vi "editDialog.vi"(0 "reference":refnum<class "ClassNode.lvclass">, 1 "insidePackageNode":bool, 5 "error in (no error)":errorcluster) -> (14 "reference out":refnum<class "ClassNode.lvclass">, 15 "changeConnection":T2, 16 "cancel":bool, 19 "error out":errorcluster)   [LabVIEW 2016, in "ClassNode.lvclass"]
doc: "Edit Dialog"
uses:
  <resource>/Framework/Providers/Open_GDS/UML/ClassNode_class/ClassNode.lvclass
  C:/Program Files (x86)/National Instruments/LabVIEW 2016/resource/Framework/Providers/Open_GDS/UML/AbstractNode_class/AbstractNode.lvclass
  <resource>/Framework/Providers/Open_GDS/UML/AbstractNode_class/private/NodeConnectionStatsType.ctl
  <resource>/Framework/Providers/Open_GDS/UML/UMLEditor/UMLEditor_StoredPathes.ctl
  <resource>/Framework/Providers/Open_GDS/ClassProviders/Common/CommonVIs/CommonVIs_StereoType.ctl
  <resource>/Framework/Providers/Open_GDS/UML/ContextHelp/ContextHelp_HelpTexts.ctl
  <resource>/Framework/Providers/Open_GDS/UML/MultiLineString_class/MultiLineString.lvclass
  <resource>/Framework/Providers/Open_GDS/UML/AbstractNode_class/AbstractNode.lvclass
  <resource>/Framework/Providers/Open_GDS/UML/Graph_class/Graph.lvclass
panel:
  in  "Class owner":u16(ring) items=["<No owner>", "FalconRocket", "RocketEngineBase", "SimulatedRocket", "TempSensor", "TestSystem"]
  out "RelText":string="Relative path used"
  out "UserText":string="When creating an enum-type just state the different enumeration members in a list like this:\nE.g.\nElement 1\nElement 2\n\nE.g.\nVolt(V)\nCurrent(A)\nResistance(ohm)\n"
  in  "ShowAttrib":bool caption="Show Attributes"
  in  "ShowMethods":bool caption="Show Methods"
  in  "Help":bool
  in  "AddMethod":bool
  in  "AddAttribute":bool
  in  "Stereo Type":T1(ring)=enum."ENUM"
  in  "Class Name":string
  in  "ClassPath":path caption="LvClassPath(Optional)"
  in  "Attribute":string
  in  "Methods":string
  in  "connection":bool caption="Connect to Package"
  in  "Cancel Button":bool
  in  "OK Button":bool
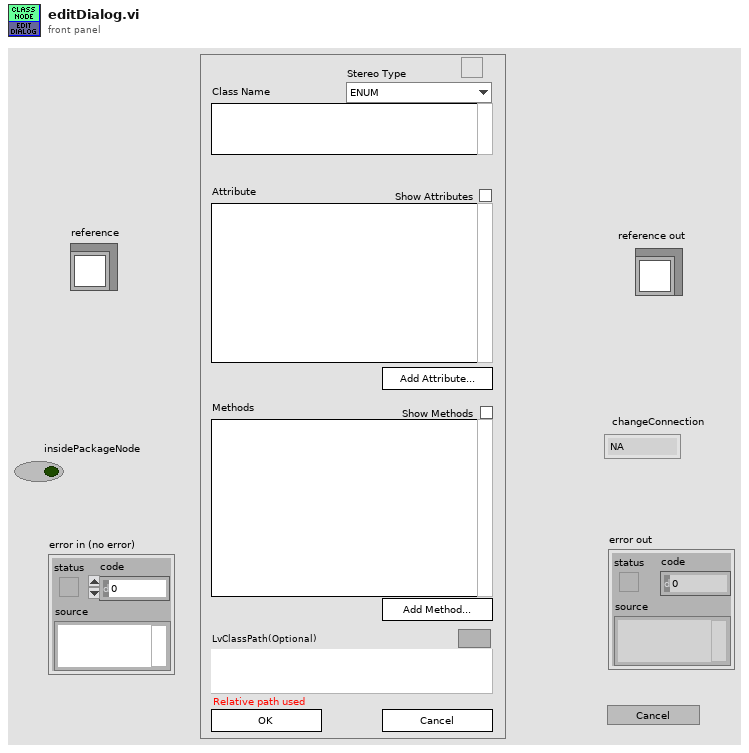
[diagram p1: front panel]
types:
  T1 = enum16{"None", "TYPE", "ENUM", "ABSTRACT", "ACTOR", "GUI", "SINGLETON", "SIGNAL", "BOUNDARY", "ENTITY", "CONTROL", "LEGACY", "APPLICATION", "VI", "LVLIB"}
  T2 = typedef "AbstractNode.lvclass/NodeConnectionStatsType.ctl" = enum16{"NA", "Connect", "DisConnect"}
  T3 = typedef "CommonVIs_StereoType.ctl" = enum16{"None", "TYPE", "ENUM", "ABSTRACT", "ACTOR", "GUI", "SINGLETON", "SIGNAL", "BOUNDARY", "ENTITY", "CONTROL", "LEGACY", "APPLICATION", "VI", "LVLIB"}
  T4 = typedef "UMLEditor_StoredPathes.ctl" = enum16{"LastSearchPath", "QueuedArrayStateVI", "ClassBasePath", "ViTemplatePath", "ApplicationTemplatePath", "IniFilePath", "WizDir", "RevPlugInPath"}
  T5 = enum32{"existing file", "new file", "new or existing file", "existing dir", "new dir", "new or existing dir", "existing file (use LLBs)", "new file (use LLBs)", "new or existing file (use LLBs)", "new or existing file or directory (use LLBs)"}
  T6 = enum16{"None", "TYPE", "ENUM", "GUI", "SINGLETON", "SIGNAL", "BOUNDARY", "ENTITY", "CONTROL", "LEGACY", "APPLICATION", "VI", "LVLIB"}
  T7 = typedef "ContextHelp_HelpTexts.ctl" = enum16{"None(Hide)", "Default", "Help", "Welcome", "GettingStarted", "ClassDiagram_Help", "SequenceDiagram_Help", "UseCaseDiagram_Help", "BSelect", "BClass", "BInterface", "BPackage", "BNote", "BDependency", "BInheritance", "BInterfaceImplementation", "BAssociation", "BAggregation", "BCompAggregation", "BNoteConnector", "BObject", "BActionBar", "BCall", "BSystem", "BActor", "BUseCase", "BGeneralization", "BIncludes", "BExtends", "BUseCaseDiagramAssociation", "ClassRelationshipEdge editDialog_Bent Style", "ClassRelationshipEdge editDialog_RelationType", "ClassRelationshipEdge editDialog_Reverse association", "ClassRelationshipEdge editDialog_Start label", "ClassRelationshipEdge editDialog_Middle label", "ClassRelationshipEdge editDialog_End label", "UMLEditor reversedEngineering_Pathes", "ReversedEngineering StateReverseDialog_Help", "ReversedEngineering StateQueuedSettings_Help", "UMLEditor reversedEngineering_AddTopVIs", "UMLEditor reversedEngineering_AddClasses", "UMLEditor reversedEngineering_AddDirs", "UMLEditor reversedEngineering_Recursively", "UMLEditor reversedEngineering_Remove", "UMLEditor reversedEngineering_ClearList", "UMLEditor reversedEngineering_HideSubAss", "UMLEditor reversedEngineering_CreateTypes", "UMLEditor reversedEngineering_OnlyInheritance", "UMLEditor reversedEngineering_CreateApplication", "UMLEditor reversedEngineering_OK", "UMLEditor reversedEngineering_Cancel", "UMLEditor reversedEngineering_Help", "UMLEditor createWizardScriptFile_ScriptfilePath", "UMLEditor createWizardScriptFile_ClassPath", "UMLEditor createWizardScriptFile_Use", "UMLEditor createWizardScriptFile_PrivateDirName", "UMLEditor createWizardScriptFile_DirAppend", "UMLEditor createWizardScriptFile_Separator Character", "UMLEditor createWizardScriptFile_OK", "UMLEditor createWizardScriptFile_Cancel", "UMLEditor createWizardScriptFile_Help", "ClassNode editDialog_Class Name", "InterfaceNode editDialog_Class Name", "ClassNode editDialog_Attribute", "ClassNode editDialog_Methods", "InterfaceNode editDialog_Methods", "ClassNode editDialog_connection", "InterfaceNode editDialog_connection", "ClassNode editDialog_StereoType", "ClassNode editDialog_ShowAttrib", "ClassNode editDialog_ShowMethods", "ClassNode editDialog_ClassPath", "ClassNode editDialog_AddAttribute", "ClassNode editDialog_AddMethod", "InterfaceNode editDialog_AddMethod", "ClassNode AttributeGuide_AttributeName", "ClassNode AttributeGuide_Array?", "ClassNode AttributeGuide_Data Type", "ClassNode AttributeGuide_RefName", "ClassNode AttributeGuide_Preview", "ClassNode AttributeGuide_OK", "ClassNode AttributeGuide_Cancel", "ClassNode MethodGuide_Visibility", "ClassNode MethodGuide_Method Name", "ClassNode MethodGuide_Preview", "ClassNode MethodGuide_OK", "ClassNode MethodGuide_Cancel", "CallNode EditCallProperties_AllButtons", "ObjectNode EditObjectlProperties_AllButtons", "ActorNode EditActorProperties_AllButtons", "UseCaseRelationshipNode EditUseCaselProperties_AllButtons", "UseCaseNode EditUseCaselProperties_AllButtons", "SystemNode EditSystemProperties_AllButtons", "ReversedEngineering UpdateAttributes_AllButtons", "StateNode editDialog_AllButtons", "StateTransition editDialog_AllButtons", "ArrangeNodes Main_Picture", "ArrangeNodes Main_Zoom", "ArrangeNodes Main_Auto Zoom", "ArrangeNodes Main_shorten", "ArrangeNodes Main_Min Length", "ArrangeNodes Main_Max Length", "ArrangeNodes Main_increase", "ArrangeNodes Main_decrease", "ArrangeNodes Main_Shake", "ArrangeNodes Main", "BState", "BInitialState", "BFinalState", "BStateTransition", "StateDiagram_Help", "StateDiagram_PropertiesAllButtons", "ReversedEngineering StateReverseDialog_ClearStates", "ReversedEngineering StateReverseDialog_UseQueuedStateMachines", "ReversedEngineering StateReverseDialog_QueuedSettings", "ReversedEngineering StateReverseDialog_SearchForVIs", "ReversedEngineering StateReverseDialog_SearchCriteria", "OptionsDialog_ClassBasePath", "OptionsDialog_VIPath", "OptionsDialog_ApplicationPath", "OptionsDialog_WizDir", "OptionsDialog_IniFilePath", "OptionsDialog_DefineColors", "OptionsDialog_Help", "OptionsDialog_CreateTypes", "ClassRelationshipEdge editDialog_SplitWire"}
  T8 = cluster{"Selection Start":u32, "Selection End":u32}
  T9 = typedef "ClassNode.lvclass/ObjectAttributes.ctl" = cluster{"midHeight":dbl, "botHeight":dbl, "name":refnum<class "MultiLineString.lvclass">, "attributes":refnum<class "MultiLineString.lvclass">, "methods":refnum<class "MultiLineString.lvclass">, "DEFAULT_COMPARTMENT_HEIGHT":i32, "DEFAULT_WIDTH":i32, "DEFAULT_HEIGHT":i32, "showMethods":bool, "showAttributes":bool, "ClassPath":path}
  T10 = typedef "AbstractNode.lvclass/ObjectAttributes.ctl" = cluster{"parent":refnum<class "AbstractNode.lvclass">, "children":refnum<class "AbstractNode.lvclass">[], "Hidden":bool}
  T11 = typedef "ContextHelp_ShowType.ctl" = cluster{"Header":string, "Picture":picture, "Text":string}
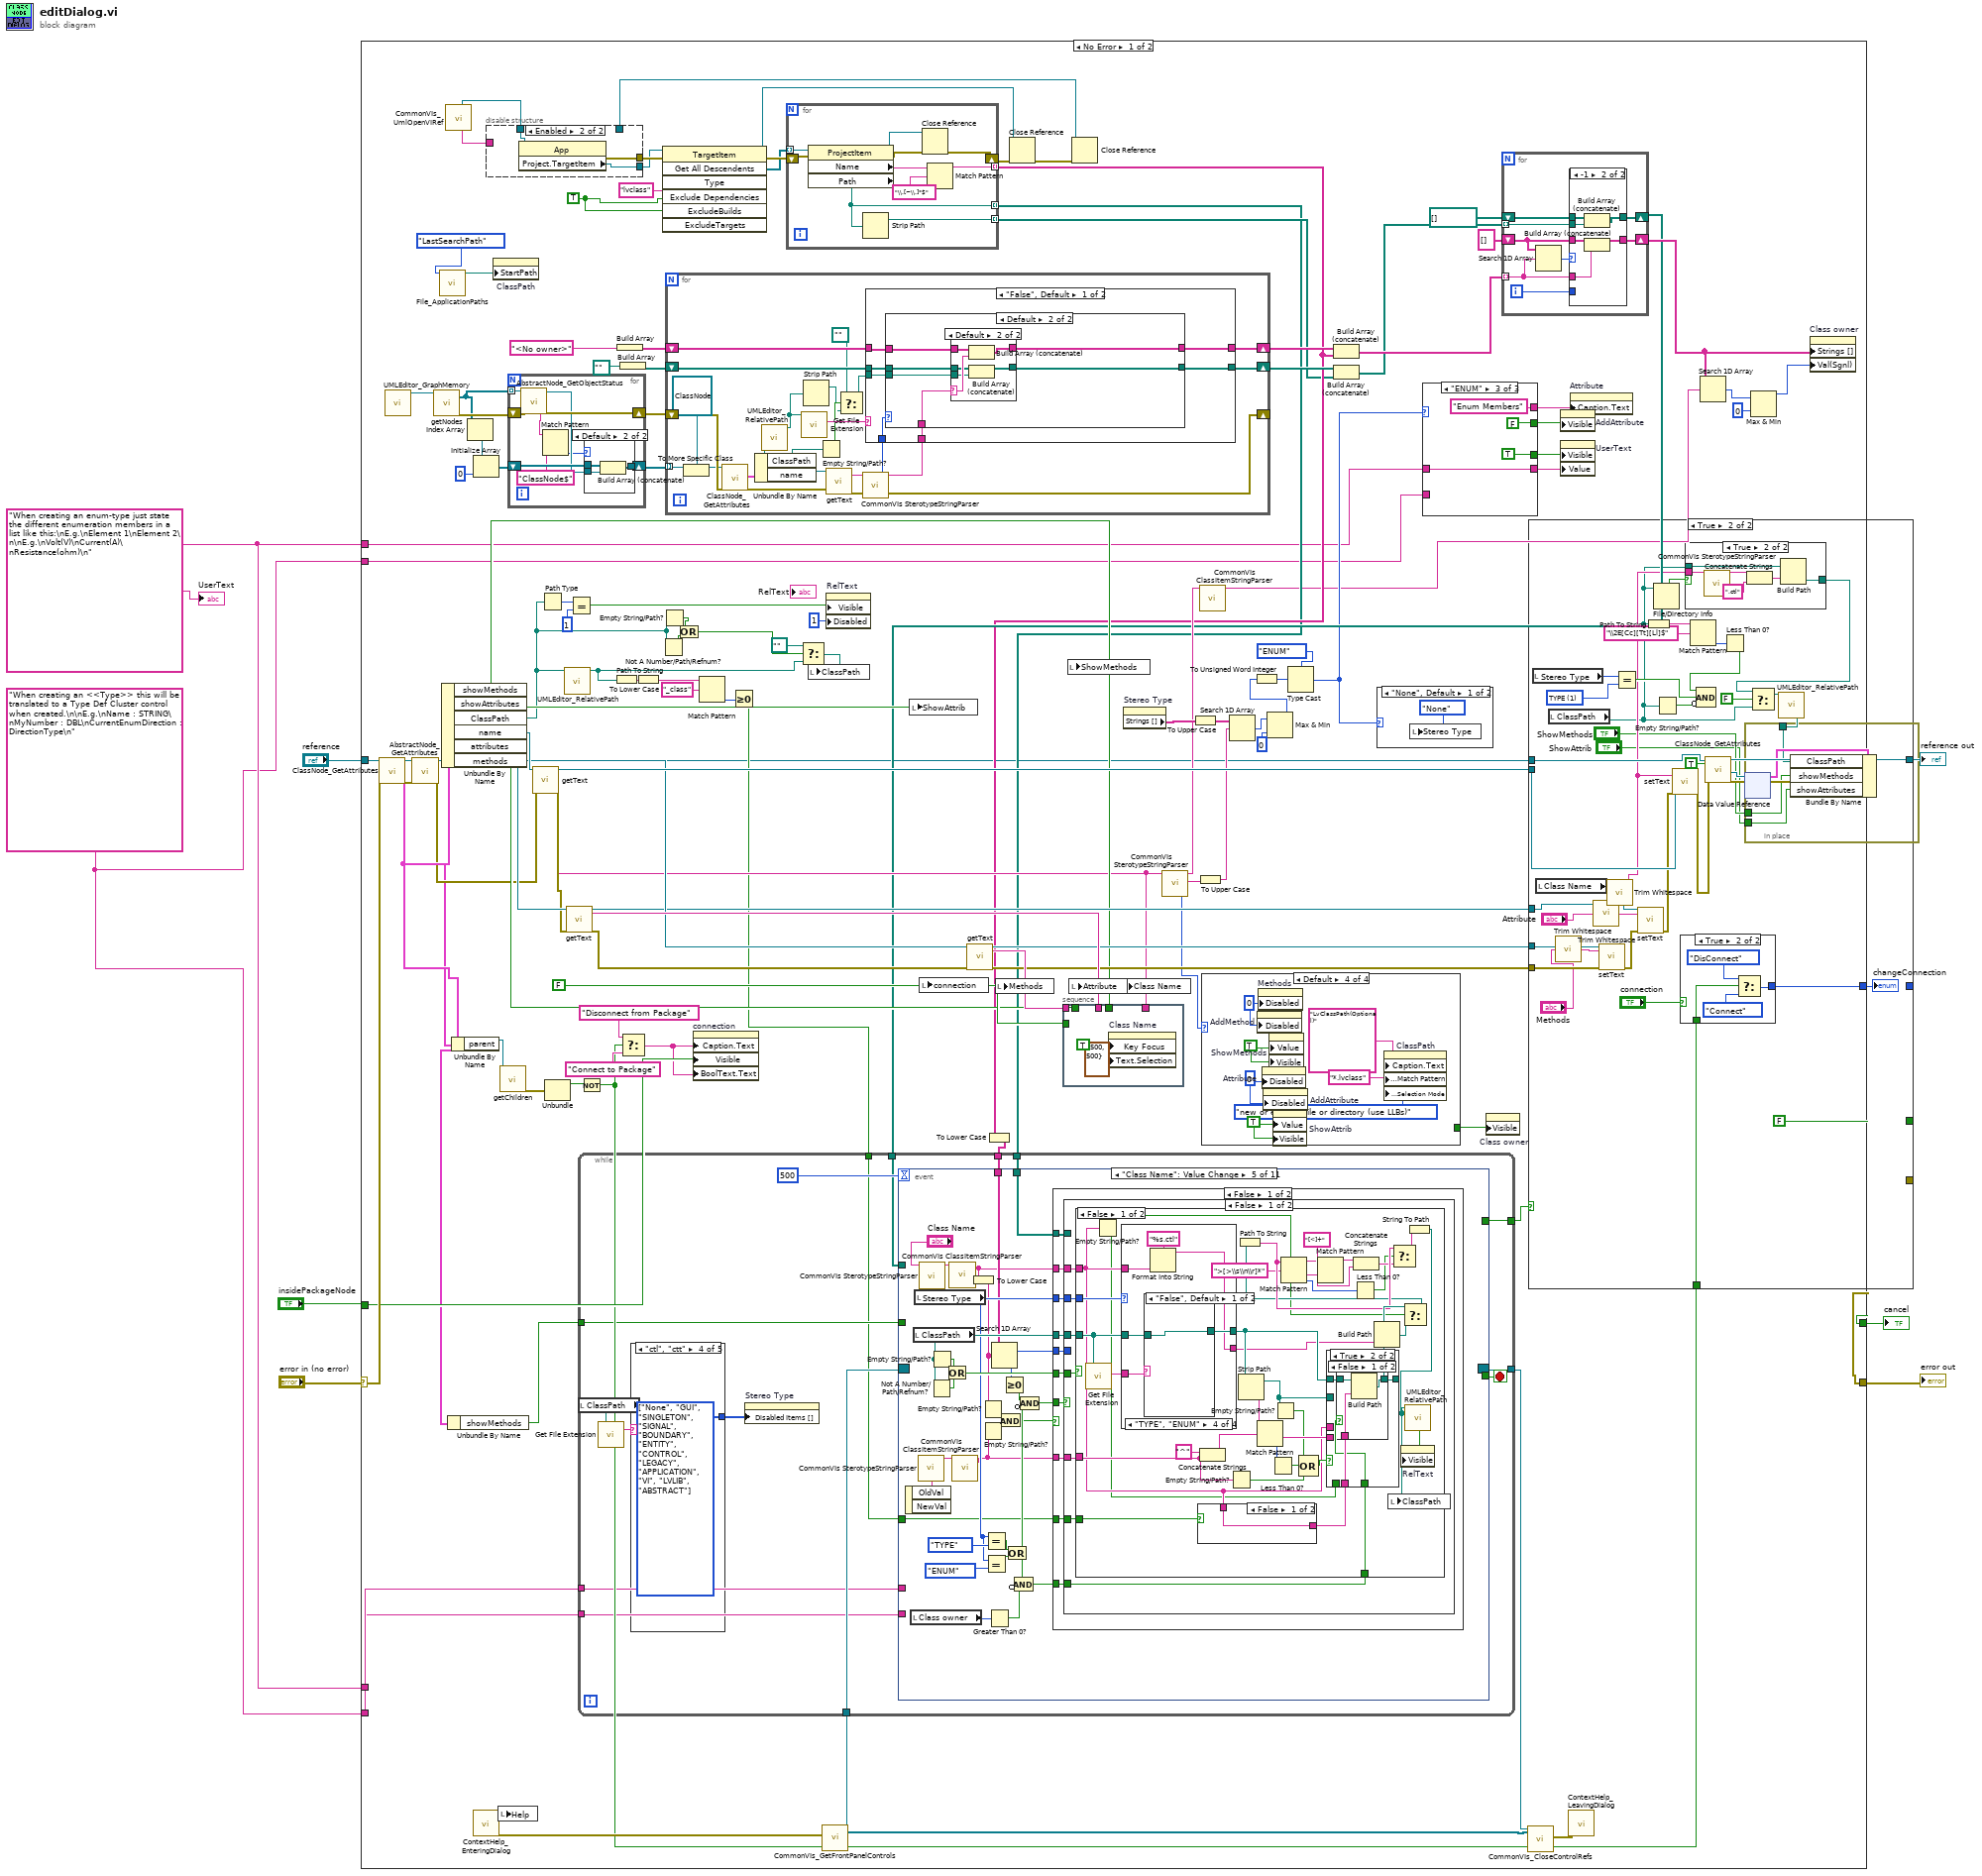
[diagram p0: block diagram]
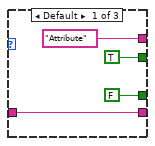
[diagram p2: hidden frame]
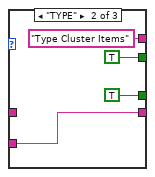
[diagram p3: hidden frame]
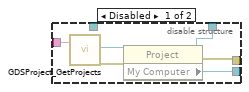
[diagram p4: hidden frame]
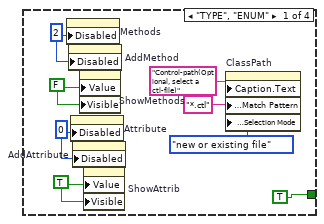
[diagram p10: hidden frame]
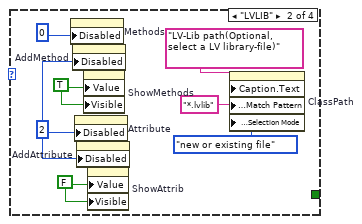
[diagram p11: hidden frame]
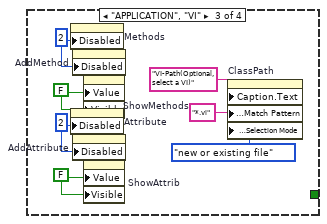
[diagram p12: hidden frame]
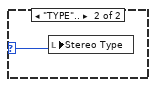
[diagram p13: hidden frame]
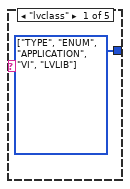
[diagram p14: hidden frame]
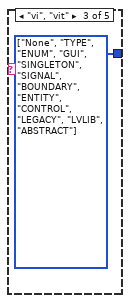
[diagram p16: hidden frame]
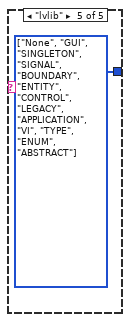
[diagram p17: hidden frame]
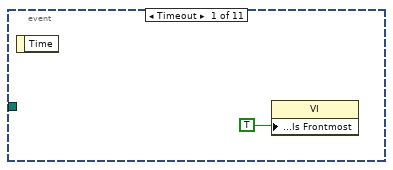
[diagram p18: hidden frame]
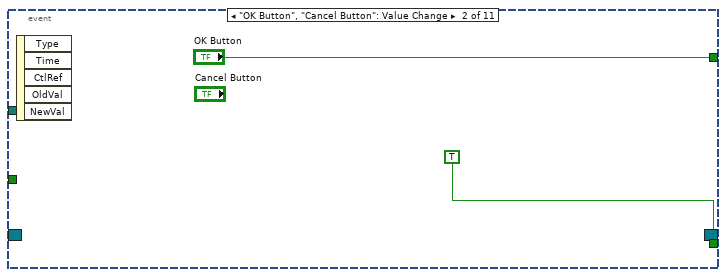
[diagram p19: hidden frame]
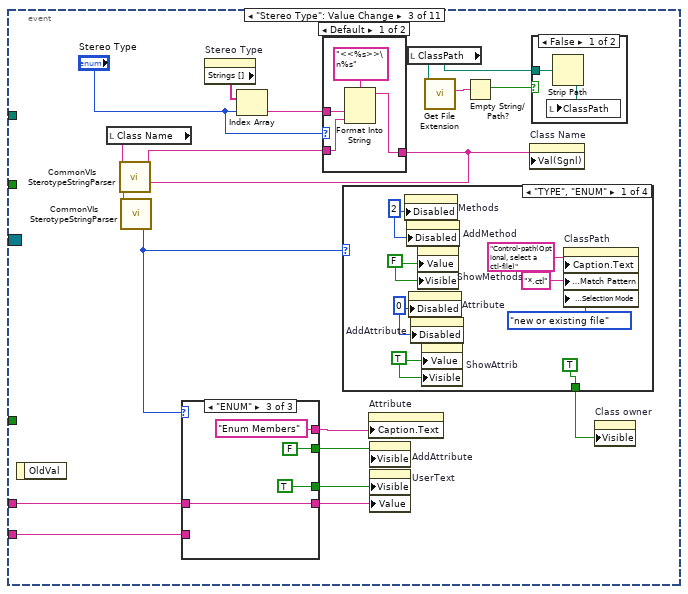
[diagram p20: hidden frame]
diagram:
  w1 = "When creating an <<Type>> this will be translated to a Type Def Cluster control when created.\n\nE.g.\nName : STRING\nMyNumber : DBL\nCurrentEnumDirection : DirectionType\n" ("UserText")
  w2 = "When creating an enum-type just state the different enumeration members in a list like this:\nE.g.\nElement 1\nElement 2\n\nE.g.\nVolt(V)\nCurrent(A)\nResistance(ohm)\n" ("UserText")
  n1 = case shown="No Error" "error in (no error)" {
    selector: "error in (no error)" -> [w128 w665]
    tunnel: "reference" -> [w129 w666]
    tunnel: [w131 w665] -> w7
    tunnel: [w130 w666] -> w6
    tunnel: "insidePackageNode" -> [w113 _]
    tunnel: [w111 _] -> w4
    tunnel: [w110 TRUE ("Key Focus")] -> w3
    tunnel: w2 -> [w18 _]
    tunnel: w1 -> [w17 _]
    tunnel: w2 -> [w25 _]
    tunnel: w1 -> [w24 _]
    frame No Error {
      w51 = TRUE ("ExcludeDependencies")
      w112 = FALSE ("connection")
      n2 = call <resource>:"ClassNode_GetAttributes.vi"("reference in"=w129, "error in (no error)"=w128) -> ("reference out"=w14:refnum<class "ClassNode.lvclass">, "Data"=w15:T9, "error out"=w13:errorcluster)  [unwired: 1 in, 14 out]
      n3 = call <resource>:"UMLEditor_GraphMemory.vi"() -> ("GraphOut"=w77:refnum<class "Graph.lvclass">)  [unwired: 2 in, 17 out]
      n4 = call <resource>:"AbstractNode_GetAttributes.vi"("reference in"=w14, "error in (no error)"=w13) -> ("reference out"=w11:refnum<class "ClassNode.lvclass">, "Data"=w10:T10, "error out"=w12:errorcluster)  [unwired: 14 in, 1 out]
      n5 = call-dynamic "getNodes.vi"("reference"=w77) -> ("nodes"=w76:refnum<class "AbstractNode.lvclass">[], "error out"=w81:errorcluster)  [unwired: 16 in, 1 out]
      n6 = call <resource>:"File_ApplicationPaths.vi"("PathName"=UMLEditor_StoredPathes."LastSearchPath" ("UMLPathes")) -> ("Path Out"=w88:path)  [unwired: 3 in, 15 out]
      n7 = Unbundle By Name(w15) -> ("showMethods"=w108:bool, "showAttributes"=w109:bool, "ClassPath"=w48:path, "name"=w125:refnum<class "MultiLineString.lvclass">, "attributes"=w124:refnum<class "MultiLineString.lvclass">, "methods"=w121:refnum<class "MultiLineString.lvclass">)
      n8 = call <resource>:"CommonVIs_UmlOpenVIRef.vi"() -> ("ProjectNameOut"=w71:string, "AppRefOut"=w32:refnum<vi>)  [unwired: 4 in, 6 out]
      n9 = Unbundle By Name(w15) -> ("showMethods"=w102:bool)
      n10 = Unbundle By Name(w10) -> ("parent"=w35:refnum<class "AbstractNode.lvclass">)
      n11 = Index Array(array=w76) -> (element=w80:refnum<class "AbstractNode.lvclass">)  [unwired: 1 in]
      n12 = Initialize Array(w80, 0 ("dimension size")) -> (w78:refnum<class "AbstractNode.lvclass">[])
      n13 = call <resource>:"ContextHelp_EnteringDialog.vi"() -> ("HelpStatus"=w101:bool, "error out"=w98:errorcluster)  [unwired: 3 in, 15 out]
      n14 = disable-structure shown="Enabled" {
        disable-tunnel: w71 -> [w147 _]
        disable-tunnel: [w146 w150] -> w69
        disable-tunnel: [w145 w151] -> w68
        disable-tunnel: [w144 _] -> w61
        disable-tunnel: w32 -> [_ w152]
        frame Disabled {
          n15 = call <resource>:"GDSProject_GetProjects.vi"("GetProjectRefByName"=w147) -> ("Project Refnum"=w149:refnum<vi>, "error out"=w148:errorcluster)  [unwired: 2 in, 15 out]
          n16 = property class="Project"(reference=w149, error in=w148) -> (reference out=w144:refnum<vi>, error out=w146:errorcluster, "My Computer"=w145:refnum<vi>)
        }
        frame Enabled {
          n17 = property class="App"(reference=w152) -> (error out=w150:errorcluster, "Project.TargetItem"=w151:refnum<vi>)  [unwired: 1 in, 1 out]
        }
      }
      n18 = property on="ClassPath" class="Path"("StartPath"=w88) -> ()  [unwired: 2 in, 2 out]
      n19 = local write "Help"(w101) -> ()
      n20 = call-dynamic "getChildren.vi"("reference"=w35) -> ("error out"=w37:errorcluster)  [unwired: 15 in, 3 out]
      n21 = for {
        shift-right: [w232] -> w74
        shift-left: w81 -> [w234]
        tunnel: w76 -> [w233] mode=indexing
        shift-right: [w229] -> w75
        shift-left: w78 -> [w231]
        n22 = call <resource>:"AbstractNode_GetObjectStatus.vi"("reference in"=w233, "error in (no error)"=w234) -> ("Class name"=w226:string, "reference out"=w230:refnum<class "AbstractNode.lvclass">, "error out"=w232:errorcluster)  [unwired: 15 out]
        n23 = Match Pattern(string=w226, regular expression="ClassNode$") -> (offset past match=w227:i32)  [unwired: 4 out]
        n24 = case shown="Default" w227 {
          tunnel: w231 -> [w235 w238]
          tunnel: w230 -> [_ w237]
          tunnel: [w235 w236] -> w229
          frame -1 {
          }
          frame Default {
            n25 = Build Array (concatenate)(w238, w237) -> (w236:refnum<class "AbstractNode.lvclass">[])
          }
        }
      }
      n26 = call-dynamic "getText.vi"("reference"=w125, "error in (no error)"=w12) -> ("reference out"=w127:refnum<class "MultiLineString.lvclass">, "text"=w107:string, "error out"=w120:errorcluster)  [unwired: 15 in]
      n27 = Path Type(1:w48) -> (0:w93:i16)
      n28 = Unbundle(w37) -> ("status"=w36:bool)  [unwired: 2 out]
      n29 = call <resource>:"UMLEditor_RelativePath.vi"("Path In"=w48) -> ("ConvertToAbsolutePath(If possible)"=w31:path)  [unwired: 1 in, 17 out]
      n30 = call-dynamic "getText.vi"("reference"=w124, "error in (no error)"=w120) -> ("reference out"=w118:refnum<class "MultiLineString.lvclass">, "text"=w123:string, "error out"=w119:errorcluster)  [unwired: 15 in]
      n31 = Equal?(x=w93, y=i16 1) -> (x = y?=w91:bool)
      n32 = Not(x=w36) -> (.not. x?=w34:bool)
      n33 = Path To String(path=w31) -> (string=w30:string)
      n34 = Build Array("<No owner>") -> (w72:string[])
      n35 = Build Array(path "" ("ClassPath")) -> (w60:path[])
      n36 = Select(t="Disconnect from Package", s=w34, f="Connect to Package") -> (s? t:f=w33:string)
      n37 = To Lower Case(string=w30) -> (all lower case string=w28:string)
      n38 = Not A Number/Path/Refnum?(number/path/refnum=w48) -> (NaN/Path/Refnum?=w50:bool)
      n39 = Empty String/Path?(string/path=w48) -> (empty?=w49:bool)
      n40 = invoke class="TargetItem" method="Get All Descendents"(reference=w68, error in=w69, "Type"="lvclass", "Exclude Dependencies"=w51, "ExcludeBuilds"=w51) -> (reference out=w64:refnum<vi>, error out=w66:errorcluster, "All Descendents"=w63:refnum<vi>[])  [unwired: 2 in, 4 out]
      n41 = for {
        tunnel: w75 -> [w182] mode=indexing
        shift-right: [w189] -> _
        shift-left: w74 -> [w200]
        shift-right: [w194] -> w67
        shift-left: w72 -> [w195]
        shift-right: [w190] -> w59
        shift-left: w60 -> [w191]
        n42 = To More Specific Class(target class=refnum<class "ClassNode.lvclass"> refnum ("reference in"), reference=w182) -> (specific class reference=w180:refnum<class "ClassNode.lvclass">)  [unwired: 1 in, 1 out]
        n43 = call <resource>:"ClassNode_GetAttributes.vi"("reference in"=w180, "error in (no error)"=w200) -> ("Data"=w179:T9, "error out"=w198:errorcluster)  [unwired: 1 in, 15 out]
        n44 = Unbundle By Name(w179) -> ("ClassPath"=w187:path, "name"=w199:refnum<class "MultiLineString.lvclass">)
        n45 = call <resource>:"UMLEditor_RelativePath.vi"("Path In"=w187) -> ("ConvertToAbsolutePath(If possible)"=w188:path)  [unwired: 1 in, 17 out]
        n46 = call <vilib>:"Get File Extension.vi"("file"=w188) -> ("lowercase file extension"=w196:string)  [unwired: 1 in, 9 out]
        n47 = Strip Path(path=w188) -> (stripped path=w185:path)  [unwired: 1 out]
        n48 = Empty String/Path?(string/path=w187) -> (empty?=w186:bool)
        n49 = call-dynamic "getText.vi"("reference"=w199, "error in (no error)"=w198) -> ("text"=w197:string, "error out"=w189:errorcluster)  [unwired: 15 in, 1 out]
        n50 = Select(t=path "", s=w186, f=w185) -> (s? t:f=w184:path)
        n51 = call <resource>:"CommonVIs SterotypeStringParser.vi"("SterotypeStringIn"=w197) -> ("StereoType"=w193:T3, "Name"=w192:string)  [unwired: 17 out]
        n52 = case shown="\"False\", Default" w196 {
          tunnel: w195 -> [w206 w225]
          tunnel: [w207 w225] -> w194
          tunnel: w193 -> [w205 _]
          tunnel: w192 -> [w204 _]
          tunnel: w191 -> [w203 w224]
          tunnel: [w202 w224] -> w190
          tunnel: w184 -> [w201 _]
          frame "False", Default {
            n53 = case shown="Default" w205 {
              tunnel: [w209 w215] -> w207
              tunnel: w206 -> [w209 w214]
              tunnel: w204 -> [_ w213]
              tunnel: w203 -> [w208 w212]
              tunnel: [w208 w211] -> w202
              tunnel: w201 -> [_ w210]
              frame "TYPE", "ENUM", "APPLICATION".."LVLIB" {
              }
              frame Default {
                n54 = case shown="Default" w213 {
                  selector: w213 -> [_ w222]
                  tunnel: [w217 w221] -> w215
                  tunnel: w214 -> [w217 w223]
                  tunnel: w212 -> [w216 w220]
                  tunnel: [w216 w219] -> w211
                  tunnel: w210 -> [_ w218]
                  frame "" {
                  }
                  frame Default {
                    n55 = Build Array (concatenate)(w223, w222) -> (w221:string[])
                    n56 = Build Array (concatenate)(w220, w218) -> (w219:path[])
                  }
                }
              }
            }
          }
          frame "ctl", "ctt", "vi", "vit" {
          }
        }
      }
      n57 = Or(x=w49, y=w50) -> (x .or. y?=w47:bool)
      n58 = property on="connection" class="Bool (strict)"("Caption.Text"=w33, "Visible"=w113, "BoolText.Text"=w33) -> ()  [unwired: 2 in, 2 out]
      n59 = Match Pattern(string=w28, regular expression="_class") -> (offset past match=w27:i32)  [unwired: 1 in, 3 out]
      n60 = Greater Or Equal To 0?(x=w27) -> (x >= 0?=w26:bool)
      n61 = for {
        tunnel: w63 -> [w178] mode=indexing
        tunnel: [w175] -> w41 mode=indexing
        shift-right: [w171] -> w65
        shift-left: w66 -> [w172]
        tunnel: [w170] -> w39 mode=indexing
        tunnel: [w169] -> w38 mode=indexing
        n62 = property class="ProjectItem"(reference=w178, error in=w172) -> (reference out=w173:refnum<vi>, error out=w174:errorcluster, "Name"=w177:string, "Path"=w169:path)
        n63 = Strip Path(path=w169) -> (stripped path=w170:path)  [unwired: 1 out]
        n64 = Close Reference(reference=w173, error in (no error)=w174) -> (error out=w171:errorcluster)
        n65 = Match Pattern(string=w177, regular expression="\\.[~\\.]*$") -> (before substring=w175:string)  [unwired: 4 out]
      }
      n66 = Select(t=path "", s=w47, f=w31) -> (s? t:f=w90:path)
      n67 = local write "ClassPath"(w90) -> ()
      n68 = call <resource>:"CommonVIs_GetFrontPanelControls.vi"("error in (no error)"=w98) -> ("Event Registration Refnum"=w97:refnum<event-registration>, "ControlRefs"=w100:refnum<vi>[])  [unwired: 1 in, 16 out]
      n69 = property on="RelText" class="Str"("Visible"=w91, "Disabled"=u8 1) -> ()  [unwired: 2 in, 2 out]
      n70 = local write "ShowAttrib"(w109) -> ()
      n71 = local write "connection"(w112) -> ()
      n72 = call-dynamic "getText.vi"("reference"=w121, "error in (no error)"=w119) -> ("reference out"=w117:refnum<class "MultiLineString.lvclass">, "text"=w122:string, "error out"=w116:errorcluster)  [unwired: 15 in]
      n73 = To Lower Case(string=w41) -> (all lower case string=w44:string[])
      n74 = local write "Methods"(w122) -> ()
      n75 = Close Reference(reference=w64, error in (no error)=w65) -> (error out=w62:errorcluster)
      n76 = stacked-sequence {
        tunnel: w107 -> [_]
        tunnel: w122 -> [_]
        tunnel: w112 -> [_]
        tunnel: w123 -> [_]
        tunnel: w109 -> [_]
        tunnel: w108 -> [_]
        frame #0 {
          n77 = property on="Class Name" class="Str"("Key Focus"=TRUE, "Text.Selection"=T8 {"Selection Start"=500, "Selection End"=500}) -> ()  [unwired: 2 in, 2 out]
        }
      }
      n78 = local write "ShowMethods"(w108) -> ()
      n79 = local write "Attribute"(w123) -> ()
      n80 = Close Reference(reference=w61, error in (no error)=w62) -> ()  [unwired: 1 out]
      n81 = local write "Class Name"(w107) -> ()
      n82 = property on="Stereo Type" class="Enum (strict)"() -> ("Strings []"=w105:string[])  [unwired: 2 in, 2 out]
      n83 = call <resource>:"CommonVIs SterotypeStringParser.vi"("SterotypeStringIn"=w107) -> ("StereoType"=w95:T3, "Name"=w58:string, "Sterotype"=w106:string)  [unwired: 16 out]
      n84 = To Upper Case(1:w105) -> (0:w104:string[])
      n85 = To Upper Case(1:w106) -> (0:w103:string)
      n86 = call <resource>:"CommonVIs ClassItemStringParser.vi"("ClassItemNameIn"=w58) -> ("Class"=w16:string)  [unwired: 18 out]
      n87 = case shown="Default" w95 {
        tunnel: [TRUE ("ShowMethods") _ _ _] -> w82
        frame "TYPE", "ENUM" {
          w243 = TRUE ("ShowMethods")
          w244 = u8 0 ("Disabled")
          w245 = FALSE ("ShowMethods")
          w246 = u8 2 ("Disabled")
          n88 = property on="Methods" class="Str"("Disabled"=w246) -> ()  [unwired: 2 in, 2 out]
          n89 = property on="AddMethod" class="Bool"("Disabled"=w246) -> ()  [unwired: 2 in, 2 out]
          n90 = property on="Attribute" class="Str"("Disabled"=w244) -> ()  [unwired: 2 in, 2 out]
          n91 = property on="AddAttribute" class="Bool"("Disabled"=w244) -> ()  [unwired: 2 in, 2 out]
          n92 = property on="ShowMethods" class="Bool (strict)"("Value"=w245, "Visible"=w245) -> ()  [unwired: 2 in, 2 out]
          n93 = property on="ShowAttrib" class="Bool (strict)"("Value"=w243, "Visible"=w243) -> ()  [unwired: 2 in, 2 out]
          n94 = property on="ClassPath" class="Path"("Caption.Text"="Control-path(Optional, select a ctl-file)", "Browse Options:Match Pattern"="*.ctl" ("Browse Dialog Options:Pattern Label"), "Browse Options:Selection Mode"=T5."new or existing file" ("Browse Dialog Options:Selection Mode")) -> ()  [unwired: 2 in, 2 out]
        }
        frame "LVLIB" {
          w251 = FALSE ("ShowMethods")
          w248 = u8 2 ("Disabled")
          w252 = TRUE ("ShowMethods")
          n95 = property on="Methods" class="Str"("Disabled"=u8 0) -> ()  [unwired: 2 in, 2 out]
          n96 = property on="AddMethod" class="Bool"("Disabled"=w248) -> ()  [unwired: 2 in, 2 out]
          n97 = property on="Attribute" class="Str"("Disabled"=w248) -> ()  [unwired: 2 in, 2 out]
          n98 = property on="AddAttribute" class="Bool"("Disabled"=w248) -> ()  [unwired: 2 in, 2 out]
          n99 = property on="ShowMethods" class="Bool (strict)"("Value"=w252, "Visible"=w252) -> ()  [unwired: 2 in, 2 out]
          n100 = property on="ShowAttrib" class="Bool (strict)"("Value"=w251, "Visible"=w251) -> ()  [unwired: 2 in, 2 out]
          n101 = property on="ClassPath" class="Path"("Caption.Text"="LV-Lib path(Optional, select a LV library-file)", "Browse Options:Match Pattern"="*.lvlib" ("Browse Dialog Options:Pattern Label"), "Browse Options:Selection Mode"=T5."new or existing file" ("Browse Dialog Options:Selection Mode")) -> ()  [unwired: 2 in, 2 out]
        }
        frame "APPLICATION", "VI" {
          w257 = FALSE ("ShowMethods")
          w259 = u8 2 ("Disabled")
          w258 = FALSE ("ShowMethods")
          w260 = u8 2 ("Disabled")
          n102 = property on="Methods" class="Str"("Disabled"=w260) -> ()  [unwired: 2 in, 2 out]
          n103 = property on="Attribute" class="Str"("Disabled"=w259) -> ()  [unwired: 2 in, 2 out]
          n104 = property on="AddMethod" class="Bool"("Disabled"=w260) -> ()  [unwired: 2 in, 2 out]
          n105 = property on="AddAttribute" class="Bool"("Disabled"=w259) -> ()  [unwired: 2 in, 2 out]
          n106 = property on="ShowMethods" class="Bool (strict)"("Value"=w258, "Visible"=w258) -> ()  [unwired: 2 in, 2 out]
          n107 = property on="ShowAttrib" class="Bool (strict)"("Value"=w257, "Visible"=w257) -> ()  [unwired: 2 in, 2 out]
          n108 = property on="ClassPath" class="Path"("Caption.Text"="VI-Path(Optional, select a VI)", "Browse Options:Match Pattern"="*.vi" ("Browse Dialog Options:Pattern Label"), "Browse Options:Selection Mode"=T5."new or existing file" ("Browse Dialog Options:Selection Mode")) -> ()  [unwired: 2 in, 2 out]
        }
        frame Default {
          w264 = TRUE ("ShowMethods")
          w266 = u8 0 ("Disabled")
          w265 = TRUE ("ShowMethods")
          w267 = u8 0 ("Disabled")
          n109 = property on="AddMethod" class="Bool"("Disabled"=w267) -> ()  [unwired: 2 in, 2 out]
          n110 = property on="Methods" class="Str"("Disabled"=w267) -> ()  [unwired: 2 in, 2 out]
          n111 = property on="Attribute" class="Str"("Disabled"=w266) -> ()  [unwired: 2 in, 2 out]
          n112 = property on="AddAttribute" class="Bool"("Disabled"=w266) -> ()  [unwired: 2 in, 2 out]
          n113 = property on="ShowMethods" class="Bool (strict)"("Value"=w265, "Visible"=w265) -> ()  [unwired: 2 in, 2 out]
          n114 = property on="ShowAttrib" class="Bool (strict)"("Value"=w264, "Visible"=w264) -> ()  [unwired: 2 in, 2 out]
          n115 = property on="ClassPath" class="Path"("Caption.Text"="LvClassPath(Optional)", "Browse Options:Match Pattern"="*.lvclass" ("Browse Dialog Options:Pattern Label"), "Browse Options:Selection Mode"=T5."new or existing file or directory (use LLBs)" ("Browse Dialog Options:Selection Mode")) -> ()  [unwired: 2 in, 2 out]
        }
      }
      n116 = Search 1D Array(1D array=w104, element=w103) -> (index of element=w84:i32)  [unwired: 1 out]
      n117 = Max & Min(x=w84, y=0) -> (max(x,y)=w83:i32)  [unwired: 1 out]
      n118 = To Unsigned Word Integer(number=w83) -> (unsigned 16bit integer=w87:u16)
      n119 = Type Cast(type=CommonVIs_StereoType."ENUM" ("StereoType"), x=w87) -> (*(type *) &x=w19:T3)
      n120 = Build Array (concatenate)(w67, w41) -> (w42:string[])
      n121 = Build Array (concatenate)(w59, w39) -> (w40:path[])
      n122 = case shown="\"None\", Default" w19 {
        selector: w19 -> [_ w269]
        frame "None", Default {
          n123 = local write "Stereo Type"(CommonVIs_StereoType."None" ("StereoType")) -> ()
        }
        frame "TYPE".. {
          n124 = local write "Stereo Type"(w269) -> ()
        }
      }
      n125 = case shown="\"ENUM\"" w19 {
        tunnel: ["Attribute" ("Caption.Text") "Type Cluster Items" ("Caption.Text") "Enum Members" ("Caption.Text")] -> w20
        tunnel: [TRUE ("Key Focus") TRUE ("Key Focus") FALSE ("Key Focus")] -> w23
        tunnel: [FALSE ("Key Focus") TRUE ("Key Focus") TRUE ("Key Focus")] -> w21
        tunnel: [w132 w136 w140] -> w22
        tunnel: w18 -> [w132 _ w140]
        tunnel: w17 -> [_ w136 _]
        frame Default {
        }
        frame "TYPE" {
        }
        frame "ENUM" {
        }
      }
      n126 = property on="Class owner" class="Ring (strict)"("Visible"=w82) -> ()  [unwired: 2 in, 2 out]
      n127 = for {
        tunnel: w42 -> [w159] mode=indexing
        shift-right: [w158] -> w54
        shift-left: string[] [] -> [w157]
        shift-right: [w155] -> w43
        shift-left: path[] [] -> [w154]
        tunnel: w40 -> [w153] mode=indexing
        i -> [w156]
        n128 = Search 1D Array(1D array=w157, element=w159) -> (index of element=w160:i32)  [unwired: 1 out]
        n129 = case shown="-1" w160 {
          tunnel: w159 -> [_ w168]
          tunnel: [w162 w166] -> w158
          tunnel: w157 -> [w162 w167]
          tunnel: w156 -> [_ _]
          tunnel: [w161 w164] -> w155
          tunnel: w154 -> [w161 w165]
          tunnel: w153 -> [_ w163]
          frame Default {
          }
          frame -1 {
            n130 = Build Array (concatenate)(w165, w163) -> (w164:path[])
            n131 = Build Array (concatenate)(w167, w168) -> (w166:string[])
          }
        }
      }
      n132 = while {
        tunnel: [w284] -> w126
        tunnel: w102 -> [w282]
        tunnel: w97 -> [w280]
        tunnel: [w279] -> w96
        tunnel: w43 -> [w275]
        tunnel: w44 -> [w274]
        tunnel: w38 -> [w273]
        tunnel: w26 -> [w272]
        tunnel: w25 -> [w271]
        tunnel: w24 -> [w270]
        stop <- w283 stop-if-true
        n133 = local read "ClassPath"() -> (w278:path)
        n134 = call <vilib>:"Get File Extension.vi"("file"=w278) -> ("lowercase file extension"=w277:string)  [unwired: 1 in, 9 out]
        n135 = case shown="\"ctl\", \"ctt\"" w277 {
          tunnel: [w285 _ w286 w287 w288] -> w276
          frame "lvclass" {
            w285 = T3[] [enum."TYPE", enum."ENUM", enum."APPLICATION", enum."VI", enum."LVLIB"] items=["None", "TYPE", "ENUM", "ABSTRACT", "ACTOR", "GUI", "SINGLETON", "SIGNAL", "BOUNDARY", "ENTITY", "CONTROL", "LEGACY", "APPLICATION", "VI", "LVLIB"] ("Disabled Items []")
          }
          frame Default {
          }
          frame "vi", "vit" {
            w286 = T3[] [enum."None", enum."TYPE", enum."ENUM", enum."GUI", enum."SINGLETON", enum."SIGNAL", enum."BOUNDARY", enum."ENTITY", enum."CONTROL", enum."LEGACY", enum."LVLIB", enum."ABSTRACT"] items=["None", "TYPE", "ENUM", "ABSTRACT", "ACTOR", "GUI", "SINGLETON", "SIGNAL", "BOUNDARY", "ENTITY", "CONTROL", "LEGACY", "APPLICATION", "VI", "LVLIB"] ("Disabled Items []")
          }
          frame "ctl", "ctt" {
            w287 = T3[] [enum."None", enum."GUI", enum."SINGLETON", enum."SIGNAL", enum."BOUNDARY", enum."ENTITY", enum."CONTROL", enum."LEGACY", enum."APPLICATION", enum."VI", enum."LVLIB", enum."ABSTRACT"] items=["None", "TYPE", "ENUM", "ABSTRACT", "ACTOR", "GUI", "SINGLETON", "SIGNAL", "BOUNDARY", "ENTITY", "CONTROL", "LEGACY", "APPLICATION", "VI", "LVLIB"] ("Disabled Items []")
          }
          frame "lvlib" {
            w288 = T3[] [enum."None", enum."GUI", enum."SINGLETON", enum."SIGNAL", enum."BOUNDARY", enum."ENTITY", enum."CONTROL", enum."LEGACY", enum."APPLICATION", enum."VI", enum."TYPE", enum."ENUM", enum."ABSTRACT"] items=["None", "TYPE", "ENUM", "ABSTRACT", "ACTOR", "GUI", "SINGLETON", "SIGNAL", "BOUNDARY", "ENTITY", "CONTROL", "LEGACY", "APPLICATION", "VI", "LVLIB"] ("Disabled Items []")
          }
        }
        n136 = property on="Stereo Type" class="Enum (strict)"("Disabled Items []"=w276) -> ()  [unwired: 2 in, 2 out]
        n137 = event shown="[4] \"Class Name\": Value Change" {
          selector: w280 -> [_ _ _ _ _ _ _ _ _ _ _]
          dyn-events: [_ _ _ _ _ _ _ _ _ _ _] -> w279
          timeout: 500 -> [_ _ _ _ _ _ _ _ _ _ _]
          tunnel: [_ "OK Button" _ FALSE ("OK Button") _ _ _ _ _ _ _] -> w284
          tunnel: [_ TRUE _ TRUE _ _ _ _ _ _ _] -> w283
          tunnel: w282 -> [_ _ _ _ _ _ _ _ _ _ _]
          tunnel: w275 -> [_ _ _ _ _ _ w526 _ _ _ _]
          tunnel: w274 -> [_ _ _ _ w372 _ _ _ _ _ _]
          tunnel: w273 -> [_ _ _ _ w367 _ _ _ _ _ _]
          tunnel: w272 -> [_ _ _ _ w366 _ _ _ _ _ _]
          tunnel: w271 -> [_ _ w293 _ _ _ _ _ _ _ _]
          tunnel: w270 -> [_ _ w292 _ _ _ _ _ _ _ _]
          event Timeout {
            n138 = event-data() -> ()  [unwired: 2 out]
            n139 = property class="VI"("Front Panel Window:Is Frontmost"=TRUE) -> ()  [unwired: 2 in, 2 out]
          }
          event "OK Button", "Cancel Button": Value Change {
            n140 = event-data() -> ()  [unwired: 6 out]
          }
          event "Stereo Type": Value Change {
            n141 = event-data() -> ()  [unwired: 2 out]
            n142 = local read "Class Name"() -> (w303:string)
            n143 = call <resource>:"CommonVIs SterotypeStringParser.vi"("SterotypeStringIn"=w303) -> ("Name"=w307:string)  [unwired: 18 out]
            n144 = property on="Stereo Type" class="Enum (strict)"() -> ("Strings []"=w308:string[])  [unwired: 2 in, 2 out]
            n145 = Index Array(array=w308, index="Stereo Type") -> (element=w302:string)
            n146 = case shown="Default" "Stereo Type" {
              tunnel: w302 -> [w354 _]
              tunnel: w307 -> [w353 w356]
              tunnel: [w352 w356] -> w300
              frame Default {
                n147 = Format Into String(format string="<<%s>>\n%s", w354, w353) -> (resulting string=w352:string)  [unwired: 2 in, 1 out]
              }
              frame "None" {
              }
            }
            n148 = call <resource>:"CommonVIs SterotypeStringParser.vi"("SterotypeStringIn"=w300) -> ("StereoType"=w296:T3)  [unwired: 18 out]
            n149 = case shown="\"ENUM\"" w296 {
              tunnel: ["Attribute" ("Caption.Text") "Type Cluster Items" ("Caption.Text") "Enum Members" ("Caption.Text")] -> w306
              tunnel: [TRUE ("Key Focus") TRUE ("Key Focus") FALSE ("Key Focus")] -> w305
              tunnel: [FALSE ("Key Focus") TRUE ("Key Focus") TRUE ("Key Focus")] -> w304
              tunnel: [w340 w344 w348] -> w294
              tunnel: w293 -> [w340 _ w348]
              tunnel: w292 -> [_ w344 _]
              frame Default {
              }
              frame "TYPE" {
              }
              frame "ENUM" {
              }
            }
            n150 = case shown="\"TYPE\", \"ENUM\"" w296 {
              tunnel: [TRUE ("ShowMethods") _ _ _] -> w295
              frame "TYPE", "ENUM" {
                w313 = TRUE ("ShowMethods")
                w314 = u8 0 ("Disabled")
                w315 = FALSE ("ShowMethods")
                w316 = u8 2 ("Disabled")
                n151 = property on="Methods" class="Str"("Disabled"=w316) -> ()  [unwired: 2 in, 2 out]
                n152 = property on="AddMethod" class="Bool"("Disabled"=w316) -> ()  [unwired: 2 in, 2 out]
                n153 = property on="Attribute" class="Str"("Disabled"=w314) -> ()  [unwired: 2 in, 2 out]
                n154 = property on="AddAttribute" class="Bool"("Disabled"=w314) -> ()  [unwired: 2 in, 2 out]
                n155 = property on="ShowMethods" class="Bool (strict)"("Value"=w315, "Visible"=w315) -> ()  [unwired: 2 in, 2 out]
                n156 = property on="ShowAttrib" class="Bool (strict)"("Value"=w313, "Visible"=w313) -> ()  [unwired: 2 in, 2 out]
                n157 = property on="ClassPath" class="Path"("Caption.Text"="Control-path(Optional, select a ctl-file)", "Browse Options:Match Pattern"="*.ctl" ("Browse Dialog Options:Pattern Label"), "Browse Options:Selection Mode"=T5."new or existing file" ("Browse Dialog Options:Selection Mode")) -> ()  [unwired: 2 in, 2 out]
              }
              frame "LVLIB" {
                w321 = FALSE ("ShowMethods")
                w318 = u8 2 ("Disabled")
                w322 = TRUE ("ShowMethods")
                n158 = property on="Methods" class="Str"("Disabled"=u8 0) -> ()  [unwired: 2 in, 2 out]
                n159 = property on="AddMethod" class="Bool"("Disabled"=w318) -> ()  [unwired: 2 in, 2 out]
                n160 = property on="Attribute" class="Str"("Disabled"=w318) -> ()  [unwired: 2 in, 2 out]
                n161 = property on="AddAttribute" class="Bool"("Disabled"=w318) -> ()  [unwired: 2 in, 2 out]
                n162 = property on="ShowMethods" class="Bool (strict)"("Value"=w322, "Visible"=w322) -> ()  [unwired: 2 in, 2 out]
                n163 = property on="ShowAttrib" class="Bool (strict)"("Value"=w321, "Visible"=w321) -> ()  [unwired: 2 in, 2 out]
                n164 = property on="ClassPath" class="Path"("Caption.Text"="LV-Lib path(Optional, select a LV library-file)", "Browse Options:Match Pattern"="*.lvlib" ("Browse Dialog Options:Pattern Label"), "Browse Options:Selection Mode"=T5."new or existing file" ("Browse Dialog Options:Selection Mode")) -> ()  [unwired: 2 in, 2 out]
              }
              frame "APPLICATION", "VI" {
                w327 = FALSE ("ShowMethods")
                w329 = u8 2 ("Disabled")
                w328 = FALSE ("ShowMethods")
                w330 = u8 2 ("Disabled")
                n165 = property on="Methods" class="Str"("Disabled"=w330) -> ()  [unwired: 2 in, 2 out]
                n166 = property on="Attribute" class="Str"("Disabled"=w329) -> ()  [unwired: 2 in, 2 out]
                n167 = property on="AddMethod" class="Bool"("Disabled"=w330) -> ()  [unwired: 2 in, 2 out]
                n168 = property on="AddAttribute" class="Bool"("Disabled"=w329) -> ()  [unwired: 2 in, 2 out]
                n169 = property on="ShowMethods" class="Bool (strict)"("Value"=w328, "Visible"=w328) -> ()  [unwired: 2 in, 2 out]
                n170 = property on="ShowAttrib" class="Bool (strict)"("Value"=w327, "Visible"=w327) -> ()  [unwired: 2 in, 2 out]
                n171 = property on="ClassPath" class="Path"("Caption.Text"="VI-Path(Optional, select a VI)", "Browse Options:Match Pattern"="*.vi" ("Browse Dialog Options:Pattern Label"), "Browse Options:Selection Mode"=T5."new or existing file" ("Browse Dialog Options:Selection Mode")) -> ()  [unwired: 2 in, 2 out]
              }
              frame Default {
                w334 = TRUE ("ShowMethods")
                w336 = u8 0 ("Disabled")
                w335 = TRUE ("ShowMethods")
                w337 = u8 0 ("Disabled")
                n172 = property on="AddMethod" class="Bool"("Disabled"=w337) -> ()  [unwired: 2 in, 2 out]
                n173 = property on="Methods" class="Str"("Disabled"=w337) -> ()  [unwired: 2 in, 2 out]
                n174 = property on="Attribute" class="Str"("Disabled"=w336) -> ()  [unwired: 2 in, 2 out]
                n175 = property on="AddAttribute" class="Bool"("Disabled"=w336) -> ()  [unwired: 2 in, 2 out]
                n176 = property on="ShowMethods" class="Bool (strict)"("Value"=w335, "Visible"=w335) -> ()  [unwired: 2 in, 2 out]
                n177 = property on="ShowAttrib" class="Bool (strict)"("Value"=w334, "Visible"=w334) -> ()  [unwired: 2 in, 2 out]
                n178 = property on="ClassPath" class="Path"("Caption.Text"="LvClassPath(Optional)", "Browse Options:Match Pattern"="*.lvclass" ("Browse Dialog Options:Pattern Label"), "Browse Options:Selection Mode"=T5."new or existing file or directory (use LLBs)" ("Browse Dialog Options:Selection Mode")) -> ()  [unwired: 2 in, 2 out]
              }
            }
            n179 = property on="Attribute" class="Str"("Caption.Text"=w306) -> ()  [unwired: 2 in, 2 out]
            n180 = property on="AddAttribute" class="Bool"("Visible"=w305) -> ()  [unwired: 2 in, 2 out]
            n181 = property on="UserText" class="Str"("Visible"=w304, "Value"=w294) -> ()  [unwired: 2 in, 2 out]
            n182 = local read "ClassPath"() -> (w297:path)
            n183 = call <vilib>:"Get File Extension.vi"("file"=w297) -> ("lowercase file extension"=w299:string)  [unwired: 1 in, 9 out]
            n184 = Empty String/Path?(string/path=w299) -> (empty?=w298:bool)
            n185 = property on="Class Name" class="Str"("Val(Sgnl)"=w300) -> ()  [unwired: 2 in, 2 out]
            n186 = case shown="False" w298 {
              tunnel: w297 -> [w339 _]
              frame False {
                n187 = Strip Path(path=w339) -> (stripped path=w338:path)  [unwired: 1 out]
                n188 = local write "ClassPath"(w338) -> ()
              }
              frame True {
              }
            }
            n189 = property on="Class owner" class="Ring (strict)"("Visible"=w295) -> ()  [unwired: 2 in, 2 out]
          }
          event Panel Close {
            n190 = event-data() -> ()  [unwired: 2 out]
          }
          event "Class Name": Value Change {
            n191 = event-data() -> ("OldVal"=w386:string)  [unwired: 2 out]
            n192 = local read "Class owner"() -> (w375:u16)
            n193 = local read "ClassPath"() -> (w385:path)
            n194 = local read "Stereo Type"() -> (w380:T1)
            n195 = call <resource>:"CommonVIs SterotypeStringParser.vi"("SterotypeStringIn"=w386) -> ("Name"=w364:string)  [unwired: 18 out]
            n196 = call <resource>:"CommonVIs SterotypeStringParser.vi"("SterotypeStringIn"="Class Name") -> ("Name"=w374:string)  [unwired: 18 out]
            n197 = Not A Number/Path/Refnum?(number/path/refnum=w385) -> (NaN/Path/Refnum?=w383:bool)
            n198 = Empty String/Path?(string/path=w385) -> (empty?=w384:bool)
            n199 = Or(x=w384, y=w383) -> (x .or. y?=w382:bool)
            n200 = call <resource>:"CommonVIs ClassItemStringParser.vi"("ClassItemNameIn"=w374) -> ("Name"=w371:string)  [unwired: 18 out]
            n201 = call <resource>:"CommonVIs ClassItemStringParser.vi"("ClassItemNameIn"=w364) -> ("Name"=w363:string)  [unwired: 18 out]
            n202 = To Lower Case(string=w371) -> (all lower case string=w362:string)
            n203 = Empty String/Path?(string/path=w362) -> (empty?=w361:bool)
            n204 = Empty String/Path?(string/path=w363) -> (empty?=w360:bool)
            n205 = Equal?(x=w380, y=T6."TYPE") -> (x = y?=w377:bool)
            n206 = Equal?(x=w380, y=T6."ENUM") -> (x = y?=w378:bool)
            n207 = Greater Than 0?(x=w375) -> (x > 0?=w376:bool)
            n208 = Search 1D Array(1D array=w372, element=w362) -> (index of element=w368:i32)  [unwired: 1 out]
            n209 = And(x=w361, y=w360) -> (x .and. y?=w359:bool)
            n210 = Greater Or Equal To 0?(x=w368) -> (x >= 0?=w370:bool)
            n211 = Or(x=w377, y=w378) -> (x .or. y?=w373:bool)
            n212 = Compound Arithmetic op=AND(w373, invert w376) -> (w365:bool)
            n213 = Compound Arithmetic op=AND(w370, invert w373) -> (w369:bool)
            n214 = case shown="False" w359 {
              tunnel: w385 -> [w397 _]
              tunnel: w382 -> [w396 _]
              tunnel: w380 -> [w395 _]
              tunnel: w371 -> [w394 _]
              tunnel: w369 -> [w393 _]
              tunnel: w368 -> [w392 _]
              tunnel: w367 -> [w391 _]
              tunnel: w366 -> [w390 _]
              tunnel: w365 -> [w389 _]
              tunnel: w363 -> [w388 _]
              frame False {
                n215 = case shown="False" w393 {
                  tunnel: w388 -> [w404 _]
                  tunnel: w397 -> [w403 _]
                  tunnel: w396 -> [w402 _]
                  tunnel: w395 -> [w401 _]
                  tunnel: w394 -> [w400 _]
                  tunnel: w392 -> [_ w502]
                  tunnel: w391 -> [_ w501]
                  tunnel: w390 -> [w399 _]
                  tunnel: w389 -> [w398 _]
                  frame False {
                    n216 = case shown="False" w402 {
                      tunnel: w401 -> [w440 _]
                      tunnel: w403 -> [w438 _]
                      tunnel: w400 -> [w408 _]
                      tunnel: w404 -> [w427 _]
                      tunnel: w399 -> [w409 _]
                      tunnel: w398 -> [w405 _]
                      frame False {
                        n217 = call <vilib>:"Get File Extension.vi"("file"=w438) -> ("lowercase file extension"=w439:string)  [unwired: 1 in, 9 out]
                        n218 = Empty String/Path?(string/path=w408) -> (empty?=w406:bool)
                        n219 = case shown="\"TYPE\", \"ENUM\"" w440 {
                          tunnel: w438 -> [w468 w477 w486 w495]
                          tunnel: w439 -> [w469 w478 w487 w496]
                          tunnel: w408 -> [w466 w475 w484 w493]
                          tunnel: [w465 w474 w483 w492] -> w432
                          tunnel: [w464 w473 w482 w491] -> w429
                          frame Default {
                            n220 = case shown="\"lvclass\"" w469 {
                              tunnel: w468 -> [w470 w472]
                              tunnel: [w470 w471] -> w465
                              frame "False", Default {
                              }
                              frame "lvclass" {
                                n221 = Strip Path(path=w472) -> (stripped path=w471:path)  [unwired: 1 out]
                              }
                            }
                            n222 = Format Into String(format string="%s.lvclass", w466) -> (resulting string=w464:string)  [unwired: 2 in, 1 out]
                          }
                          frame "APPLICATION", "VI" {
                            n223 = case shown="\"vi\"" w478 {
                              tunnel: w477 -> [w479 w481]
                              tunnel: [w479 w480] -> w474
                              frame "False", Default {
                              }
                              frame "vi" {
                                n224 = Strip Path(path=w481) -> (stripped path=w480:path)  [unwired: 1 out]
                              }
                            }
                            n225 = Format Into String(format string="%s.vi", w475) -> (resulting string=w473:string)  [unwired: 2 in, 1 out]
                          }
                          frame "LVLIB" {
                            n226 = case shown="\"lvlib\"" w487 {
                              tunnel: w486 -> [w488 w490]
                              tunnel: [w488 w489] -> w483
                              frame "False", Default {
                              }
                              frame "lvlib" {
                                n227 = Strip Path(path=w490) -> (stripped path=w489:path)  [unwired: 1 out]
                              }
                            }
                            n228 = Format Into String(format string="%s.lvlib", w484) -> (resulting string=w482:string)  [unwired: 2 in, 1 out]
                          }
                          frame "TYPE", "ENUM" {
                            n229 = case shown="\"False\", Default" w496 {
                              tunnel: w495 -> [w497 w499]
                              tunnel: [w497 w498] -> w492
                              frame "False", Default {
                              }
                              frame "ctl" {
                                n230 = Strip Path(path=w499) -> (stripped path=w498:path)  [unwired: 1 out]
                              }
                            }
                            n231 = Format Into String(format string="%s.ctl", w493) -> (resulting string=w491:string)  [unwired: 2 in, 1 out]
                          }
                        }
                        n232 = case shown="False" w409 {
                          tunnel: w408 -> [w441 w443]
                          tunnel: [w441 w442] -> w407
                          frame False {
                          }
                          frame True {
                            n233 = Concatenate Strings(w443, "_class" ("regular expression")) -> (w442:string)
                          }
                        }
                        n234 = Concatenate Strings("^" ("string"), w427) -> (w434:string)
                        n235 = Empty String/Path?(string/path=w427) -> (empty?=w423:bool)
                        n236 = Strip Path(path=w432) -> (stripped path=w428:path, name=w436:string)
                        n237 = Match Pattern(string=w436, regular expression=w434) -> (after substring=w433:string, offset past match=w426:i32)  [unwired: 3 out]
                        n238 = Less Than 0?(x=w426) -> (x < 0?=w424:bool)
                        n239 = Empty String/Path?(string/path=w428) -> (empty?=w425:bool)
                        n240 = Compound Arithmetic op=OR(w425, w424, w423) -> (w422:bool)
                        n241 = case shown="True" w422 {
                          tunnel: w432 -> [_ w459]
                          tunnel: [w448 w458] -> w431
                          tunnel: w428 -> [w449 _]
                          tunnel: w408 -> [w447 _]
                          tunnel: w433 -> [w446 _]
                          tunnel: w407 -> [_ w457]
                          tunnel: w406 -> [w445 _]
                          tunnel: w405 -> [_ w456]
                          frame False {
                            n242 = case shown="True" w445 {
                              tunnel: w449 -> [w454 w455]
                              tunnel: [w453 w455] -> w448
                              tunnel: w447 -> [w452 _]
                              tunnel: w446 -> [w451 _]
                              frame False {
                                n243 = Concatenate Strings(w452, w451) -> (w450:string)
                                n244 = Build Path(base path=w454, name or relative path=w450) -> (appended path=w453:path)
                              }
                              frame True {
                              }
                            }
                          }
                          frame True {
                            n245 = case shown="False" w456 {
                              tunnel: w459 -> [w462 w463]
                              tunnel: [w461 w463] -> w458
                              tunnel: w457 -> [w460 _]
                              frame False {
                                n246 = Build Path(base path=w462, name or relative path=w460) -> (appended path=w461:path)
                              }
                              frame True {
                              }
                            }
                          }
                        }
                        n247 = Build Path(base path=w431, name or relative path=w429) -> (appended path=w437:path)
                        n248 = Select(t=w431, s=w406, f=w437) -> (s? t:f=w411:path)
                        n249 = Path To String(path=w411) -> (string=w421:string)
                        n250 = Match Pattern(string=w421, regular expression=">[>\\s\\n\\r]*") -> (before substring=w413:string, after substring=w418:string, offset past match=w416:i32)  [unwired: 2 out]
                        n251 = Match Pattern(string=w413, regular expression="[<]+") -> (before substring=w417:string)  [unwired: 4 out]
                        n252 = Less Than 0?(x=w416) -> (x < 0?=w415:bool)
                        n253 = Concatenate Strings(w417, w418) -> (w419:string)
                        n254 = Select(t=w421, s=w415, f=w419) -> (s? t:f=w420:string)
                        n255 = String To Path(string=w420) -> (path=w410:path)
                        n256 = local write "ClassPath"(w410) -> ()
                        n257 = call <resource>:"UMLEditor_RelativePath.vi"("Path In"=w410) -> ("ConvertedToARelativePath"=w430:bool)  [unwired: 1 in, 17 out]
                        n258 = property on="RelText" class="Str"("Visible"=w430) -> ()  [unwired: 2 in, 2 out]
                      }
                      frame True {
                      }
                    }
                  }
                  frame True {
                    n259 = Index Array(array=w501, index=w502) -> (element=w500:path)
                    n260 = local write "ClassPath"(w500) -> ()
                  }
                }
              }
              frame True {
              }
            }
          }
          event "ClassPath": Value Change {
            n261 = event-data() -> ()  [unwired: 2 out]
            n262 = call <vilib>:"Get File Extension.vi"("file"="ClassPath") -> ("filename without extension"=w503:string, "lowercase file extension"=w504:string)  [unwired: 1 in, 8 out]
            n263 = case shown="Default" w504 {
              tunnel: w503 -> [_ w510 w517]
              frame Default {
                n264 = local read "Class Name"() -> (w509:string)
                n265 = property on="Class Name" class="Str"("Val(Sgnl)"=w509) -> ()  [unwired: 2 in, 2 out]
              }
              frame "ctl" {
                n266 = local read "Stereo Type"() -> (w514:T1)
                n267 = case shown="Default" w514 {
                  selector: w514 -> [_ w516]
                  tunnel: [w515 w516] -> w512
                  frame Default {
                    w515 = CommonVIs_StereoType."TYPE" ("Stereo Type")
                    n268 = local write "Stereo Type"(w515) -> ()
                  }
                  frame "TYPE", "ENUM" {
                  }
                }
                n269 = Format Into String(format string="<<%s>>\n%s", w512, w510) -> (resulting string=w511:string)  [unwired: 2 in, 1 out]
                n270 = local write "Class Name"(w511) -> ()
              }
              frame "vi", "vit" {
                n271 = local read "Stereo Type"() -> (w521:T1)
                n272 = case shown="Default" w521 {
                  selector: w521 -> [_ w523]
                  tunnel: [w522 w523] -> w519
                  frame Default {
                    w522 = CommonVIs_StereoType."VI" ("Stereo Type")
                    n273 = local write "Stereo Type"(w522) -> ()
                  }
                  frame "APPLICATION", "VI" {
                  }
                }
                n274 = Format Into String(format string="<<%s>>\n%s", w519, w517) -> (resulting string=w518:string)  [unwired: 2 in, 1 out]
                n275 = local write "Class Name"(w518) -> ()
              }
            }
            n276 = Empty String/Path?(string/path="ClassPath") -> (empty?=w506:bool)
            n277 = call <resource>:"UMLEditor_RelativePath.vi"("Path In"="ClassPath") -> ("ConvertedToARelativePath"=w507:bool)  [unwired: 1 in, 17 out]
            n278 = Compound Arithmetic op=AND(invert w506, w507) -> (w508:bool)
            n279 = property on="RelText" class="Str"("Visible"=w508) -> ()  [unwired: 2 in, 2 out]
          }
          event "Class owner": Value Change {
            n280 = event-data() -> ()  [unwired: 2 out]
            n281 = property on="Class owner" class="Ring (strict)"() -> ("Visible"=w524:bool)  [unwired: 2 in, 2 out]
            n282 = case shown="True" w524 {
              tunnel: w526 -> [_ w532]
              tunnel: "Class owner" -> [_ w531]
              frame False {
              }
              frame True {
                n283 = local read "Class Name"() -> (w541:string)
                n284 = property on="Class owner" class="Ring (strict)"() -> ("Strings []"=w537:string[])  [unwired: 2 in, 2 out]
                n285 = Index Array(array=w532, index=w531) -> (element=w527:path)
                n286 = Empty String/Path?(string/path=w527) -> (empty?=w530:bool)
                n287 = Not A Number/Path/Refnum?(number/path/refnum=w527) -> (NaN/Path/Refnum?=w529:bool)
                n288 = call <resource>:"CommonVIs SterotypeStringParser.vi"("SterotypeStringIn"=w541) -> ("Name"=w540:string, "Sterotype"=w539:string)  [unwired: 17 out]
                n289 = Index Array(array=w537, index=w531) -> (element=w536:string)
                n290 = Or(x=w530, y=w529) -> (x .or. y?=w528:bool)
                n291 = call <resource>:"CommonVIs ClassItemStringParser.vi"("ClassItemNameIn"=w540) -> ("Name"=w535:string)  [unwired: 18 out]
                n292 = case shown="True" w528 {
                  tunnel: w527 -> [w542 _]
                  frame False {
                    n293 = local write "ClassPath"(w542) -> ()
                  }
                  frame True {
                    n294 = disable-structure shown="Disabled" {
                      frame Disabled {
                        n295 = local write "ClassPath"(path "" ("ClassPath")) -> ()
                      }
                      frame Enabled {
                      }
                    }
                  }
                }
                n296 = case shown="Default" w539 {
                  selector: w539 -> [w555 _]
                  tunnel: [w556 _] -> w538
                  frame Default {
                    n297 = Format Into String(format string="<<%s>>\n", w555) -> (resulting string=w556:string)  [unwired: 2 in, 1 out]
                  }
                  frame "" {
                  }
                }
                n298 = case shown="\"\"" w535 {
                  selector: w535 -> [w544 _]
                  tunnel: [w544 "NewType"] -> w534
                  frame Default {
                  }
                  frame "" {
                  }
                }
                n299 = case shown="0, Default" w531 {
                  tunnel: w534 -> [w547 w553]
                  tunnel: w538 -> [w549 w552]
                  tunnel: [w546 w551] -> w533
                  tunnel: w536 -> [_ w550]
                  frame 0, Default {
                    n300 = Format Into String(format string="%s", initial string=w549, w547) -> (resulting string=w546:string)  [unwired: 1 in, 1 out]
                  }
                  frame 1.. {
                    n301 = Format Into String(format string="%s : %s", initial string=w552, w550, w553) -> (resulting string=w551:string)  [unwired: 1 in, 1 out]
                  }
                }
                n302 = property on="Class Name" class="Str"("Val(Sgnl)"=w533) -> ()  [unwired: 2 in, 2 out]
              }
            }
          }
          event "AddAttribute": Value Change {
            n303 = event-data() -> ()  [unwired: 4 out]
            n304 = local read "Attribute"() -> (w559:string)
            n305 = call <resource>:"AttributeGuide.vi"() -> ("Preview"=w558:string, "Canceled"=w560:bool)  [unwired: 18 out]
            n306 = case shown="False" w560 {
              tunnel: w559 -> [w566 _]
              tunnel: w558 -> [w563 _]
              frame False {
                n307 = call <vilib>:"Trim Whitespace.vi"("string"=w566) -> ("trimmed string"=w564:string)  [unwired: 1 in]
                n308 = Format Into String(format string="%s\n%s", w564, w563) -> (resulting string=w562:string)  [unwired: 2 in, 1 out]
                n309 = call <vilib>:"Trim Whitespace.vi"("string"=w562) -> ("trimmed string"=w561:string)  [unwired: 1 in]
                n310 = local write "Attribute"(w561) -> ()
              }
              frame True {
              }
            }
          }
          event "AddMethod": Value Change {
            n311 = event-data() -> ()  [unwired: 4 out]
            n312 = local read "Attribute"() -> (w573:string)
            n313 = local read "Methods"() -> (w576:string)
            n314 = call <vilib>:"Trim Whitespace.vi"("string"=w573) -> ("trimmed string"=w572:string)  [unwired: 1 in]
            n315 = Spreadsheet String To Array(delimiter (Tab)="\n", format string="%s", spreadsheet string=w572, array type (2D Dbl)=string[] [] ("Attributes")) -> (array=w568:string[])
            n316 = for {
              tunnel: w568 -> [w584] mode=indexing
              tunnel: [w580] -> w567 mode=indexing
              n317 = Match Pattern(string=w584, regular expression="^[\\s+#-]+") -> (before substring=w582:string, after substring=w581:string)  [unwired: 1 in, 2 out]
              n318 = Concatenate Strings(w582, w581) -> (w578:string)
              n319 = Match Pattern(string=w578, regular expression=":") -> (before substring=w577:string)  [unwired: 1 in, 3 out]
              n320 = call <vilib>:"Trim Whitespace.vi"("string"=w577) -> ("trimmed string"=w580:string)  [unwired: 1 in]
            }
            n321 = call <resource>:"MethodGuide.vi"("Attributes"=w567) -> ("Preview"=w575:string, "Canceled"=w574:bool)  [unwired: 17 out]
            n322 = case shown="False" w574 {
              tunnel: w576 -> [w590 _]
              tunnel: w575 -> [w587 _]
              frame False {
                n323 = call <vilib>:"Trim Whitespace.vi"("string"=w590) -> ("trimmed string"=w588:string)  [unwired: 1 in]
                n324 = Format Into String(format string="%s\n%s", w588, w587) -> (resulting string=w586:string)  [unwired: 2 in, 1 out]
                n325 = call <vilib>:"Trim Whitespace.vi"("string"=w586) -> ("trimmed string"=w585:string)  [unwired: 1 in]
                n326 = local write "Methods"(w585) -> ()
              }
              frame True {
              }
            }
          }
          event "Help": Value Change {
            n327 = event-data() -> ()  [unwired: 2 out]
            n328 = case shown="True" "Help" {
              tunnel: [ContextHelp_HelpTexts."None(Hide)" ("HelpText") ContextHelp_HelpTexts."Default" ("HelpText")] -> w592
              frame False {
              }
              frame True {
              }
            }
            n329 = call <resource>:"ContextHelp_HelpTexts.vi"("HelpText (enum or string)"=w592) -> ("HelpOut"=w593:T11)  [unwired: 18 out]
            n330 = call <resource>:"ContextHelp_SendMessageToPopUp.vi"("PopUpMessage"=w593) -> ()  [unwired: 2 in, 17 out]
          }
          event Mouse Enter {
            n331 = event-data() -> ("CtlRef"=w597:refnum<vi>)  [unwired: 1 out]
            n332 = local read "Help"() -> (w596:bool)
            n333 = call <resource>:"ContextHelp_CheckHelpForControl.vi"("Ctl Refnum"=w597, "Help"=w596) -> ()  [unwired: 1 in, 17 out]
          }
        }
      }
      n334 = call <resource>:"CommonVIs_CloseControlRefs.vi"("Event Registration Refnum"=w96, "ControlRefs"=w100) -> ("error out"=w99:errorcluster)  [unwired: 1 in, 16 out]
      n335 = case shown="True" w126 {
        tunnel: [w600 w639] -> w131
        tunnel: [w601 w638] -> w130
        tunnel: w11 -> [w601 w637]
        tunnel: w127 -> [_ w636]
        tunnel: w118 -> [_ w631]
        tunnel: w117 -> [_ w630]
        tunnel: w116 -> [w600 w629]
        tunnel: w34 -> [_ w625]
        tunnel: [enum16{"NA", "Connect", "DisConnect"}."NA" ("changeConnection") w626] -> w111
        tunnel: [TRUE ("Key Focus") FALSE ("Key Focus")] -> w110
        frame False {
        }
        frame True {
          w620 = u16 1 items=["None", "TYPE", "GUI", "SINGLETON", "SIGNAL", "BOUNDARY", "ENTITY", "CONTROL", "LEGACY"] ("StereoType")
          n336 = local read "Stereo Type"() -> (w621:T1)
          n337 = local read "Class Name"() -> (w609:string)
          n338 = local read "ClassPath"() -> (w608:path)
          n339 = call <vilib>:"Trim Whitespace.vi"("string"="Methods") -> ("trimmed string"=w622:string)  [unwired: 1 in]
          n340 = call <vilib>:"Trim Whitespace.vi"("string"="Attribute") -> ("trimmed string"=w623:string)  [unwired: 1 in]
          n341 = call-dynamic "setText.vi"("reference"=w630, "text"=w622, "error in (no error)"=w629) -> ("error out"=w632:errorcluster)  [unwired: 15 in, 1 out]
          n342 = call <vilib>:"Trim Whitespace.vi"("string"=w609) -> ("trimmed string"=w611:string)  [unwired: 1 in]
          n343 = Equal?(x=w621, y=w620) -> (x = y?=w618:bool)
          n344 = call-dynamic "setText.vi"("reference"=w631, "text"=w623, "error in (no error)"=w632) -> ("error out"=w634:errorcluster)  [unwired: 15 in, 1 out]
          n345 = Path To String(path=w608) -> (string=w614:string)
          n346 = File/Directory Info(path=w608) -> (directory=w613:bool)  [unwired: 1 in, 6 out]
          n347 = Empty String/Path?(string/path=w608) -> (empty?=w619:bool)
          n348 = call-dynamic "setText.vi"("reference"=w636, "text"=w611, "error in (no error)"=w634) -> ("error out"=w635:errorcluster)  [unwired: 15 in, 1 out]
          n349 = case shown="True" "connection" {
            tunnel: [enum16{"NA", "Connect", "DisConnect"}."NA" ("changeConnection") w660] -> w626
            tunnel: w625 -> [_ w661]
            frame False {
            }
            frame True {
              n350 = Select(t=enum16{"NA", "Connect", "DisConnect"}."DisConnect" ("changeConnection"), s=w661, f=enum16{"NA", "Connect", "DisConnect"}."Connect" ("changeConnection")) -> (s? t:f=w660:enum16{"NA", "Connect", "DisConnect"})
            }
          }
          n351 = case shown="True" w613 {
            tunnel: w608 -> [w650 w655]
            tunnel: [w645 w656] -> w612
            tunnel: w611 -> [_ w654]
            frame False {
              n352 = Strip Path(path=w650) -> (stripped path=w647:path, name=w649:string)
              n353 = Concatenate Strings(w649, ".ctl" ("string")) -> (w646:string)
              n354 = Build Path(base path=w647, name or relative path=w646) -> (appended path=w645:path)
            }
            frame True {
              n355 = call <resource>:"CommonVIs SterotypeStringParser.vi"("SterotypeStringIn"=w654) -> ("Name"=w652:string)  [unwired: 18 out]
              n356 = Concatenate Strings(w652, ".ctl" ("string")) -> (w651:string)
              n357 = Build Path(base path=w655, name or relative path=w651) -> (appended path=w656:path)
            }
          }
          n358 = Match Pattern(string=w614, regular expression="\\2E[Cc][Tt][Ll]$") -> (offset past match=w616:i32)  [unwired: 4 out]
          n359 = call <resource>:"ClassNode_GetAttributes.vi"("reference in"=w637, "OnlyGetDvrReference(False)"=TRUE, "error in (no error)"=w635) -> ("reference out"=w638:refnum<class "ClassNode.lvclass">, "DataRef"=w605:refnum<data-value>, "error out"=w639:errorcluster)  [unwired: 13 in, 1 out]
          n360 = Less Than 0?(x=w616) -> (x < 0?=w615:bool)
          n361 = Compound Arithmetic op=AND(w615, w618, invert w619) -> ()  [unwired: 1 out]
          n362 = Select(t=w612, s=FALSE, f=w608) -> (s? t:f=w610:path)
          n363 = call <resource>:"UMLEditor_RelativePath.vi"("Path In"=w610) -> ("ConvertToRelativePath(If possible)"=w604:path)  [unwired: 1 in, 17 out]
          n364 = in-place {
            in-place-border: w604 -> [w643]
            in-place-border: "ShowMethods" -> [w642]
            in-place-border: "ShowAttrib" -> [w641]
            n365 = in-place-dvr #1(w605) -> (w644:T9)  [unwired: 1 out]
            n366 = Bundle By Name(cluster=w644, "ClassPath"=w643, "showMethods"=w642, "showAttributes"=w641) -> (w640:T9)
            n367 = in-place-dvr #1(w640) -> ()  [unwired: 2 out]
          }
        }
      }
      n368 = property on="AddAttribute" class="Bool"("Visible"=w23) -> ()  [unwired: 2 in, 2 out]
      n369 = property on="UserText" class="Str"("Visible"=w21, "Value"=w22) -> ()  [unwired: 2 in, 2 out]
      n370 = call <resource>:"ContextHelp_LeavingDialog.vi"("error in (no error)"=w99) -> ()  [unwired: 2 in, 17 out]
      n371 = property on="Attribute" class="Str"("Caption.Text"=w20) -> ()  [unwired: 2 in, 2 out]
      n372 = Search 1D Array(1D array=w54, element=w16) -> (index of element=w57:i32)  [unwired: 1 out]
      n373 = Max & Min(x=w57, y=0) -> (max(x,y)=w55:i32)  [unwired: 1 out]
      n374 = property on="Class owner" class="Ring (strict)"("Strings []"=w54, "Val(Sgnl)"=w55) -> ()  [unwired: 2 in, 2 out]
    }
    frame Error {
    }
  }
  "reference out" <- w6
  "error out" <- w7
  "changeConnection" <- w4
  "cancel" <- w3
  "UserText" <- w2
